vi "Manejo de errores SubVI.vi"(8 "error in (no error)":errorcluster) -> ()   [LabVIEW 2016]
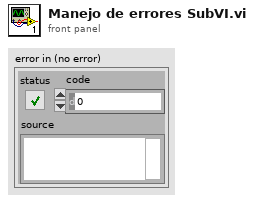
[diagram p1: front panel]
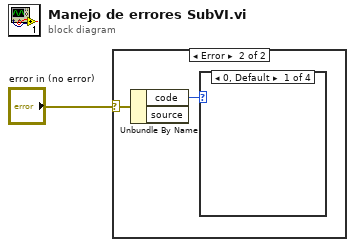
[diagram p0: block diagram]
diagram:
  n1 = case shown="Error" "error in (no error)" {
    selector: "error in (no error)" -> [_ w3]
    frame No Error {
    }
    frame Error {
      n2 = Unbundle By Name(w3) -> ("code"=w2:i32)  [unwired: 1 out]
      n3 = case shown="0, Default" w2 {
        frame 0, Default {
        }
        frame 1 {
        }
        frame 2 {
        }
        frame 3 {
        }
      }
    }
  }
